vi "CreateBeamLineChargeStateNode.vi"(8 "Error In":errorcluster, 10 "Beam Line":T1={"Type"=enum."Ion Beam Analysis", "Ion"=enum."H", "Charge State"=0, "Total Source Ion Energy (kV)"=nan} {"Charge State" min=1}, 11 "DOM Document In":refnum<k20>) -> (0 "Error out":errorcluster, 2 "Beam Line Charge State Node":refnum<k20>, 3 "DOM Document Out":refnum<k20>)   [LabVIEW 2012]
uses:
  BeamLine.ctl
  BeamLineType.ctl
  BeamLineIon.ctl
  <resource>/objmgr/DOMUserDefRef.rc
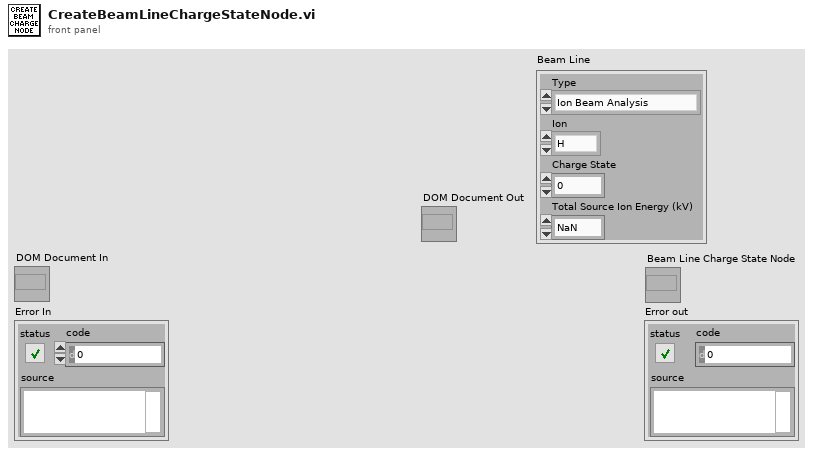
[diagram p1: front panel]
types:
  T1 = typedef "BeamLine.ctl" = cluster{"Type":T2, "Ion":T3, "Charge State":u8, "Total Source Ion Energy (kV)":dbl}
  T2 = typedef "BeamLineType.ctl" = enum16{"Ion Beam Analysis", "Auxiliary", "Radiation Damage"}
  T3 = typedef "BeamLineIon.ctl" = enum16{"H", "He", "C", "Fe", "Ni", "Pt", "Si", "Ag", "Au"}
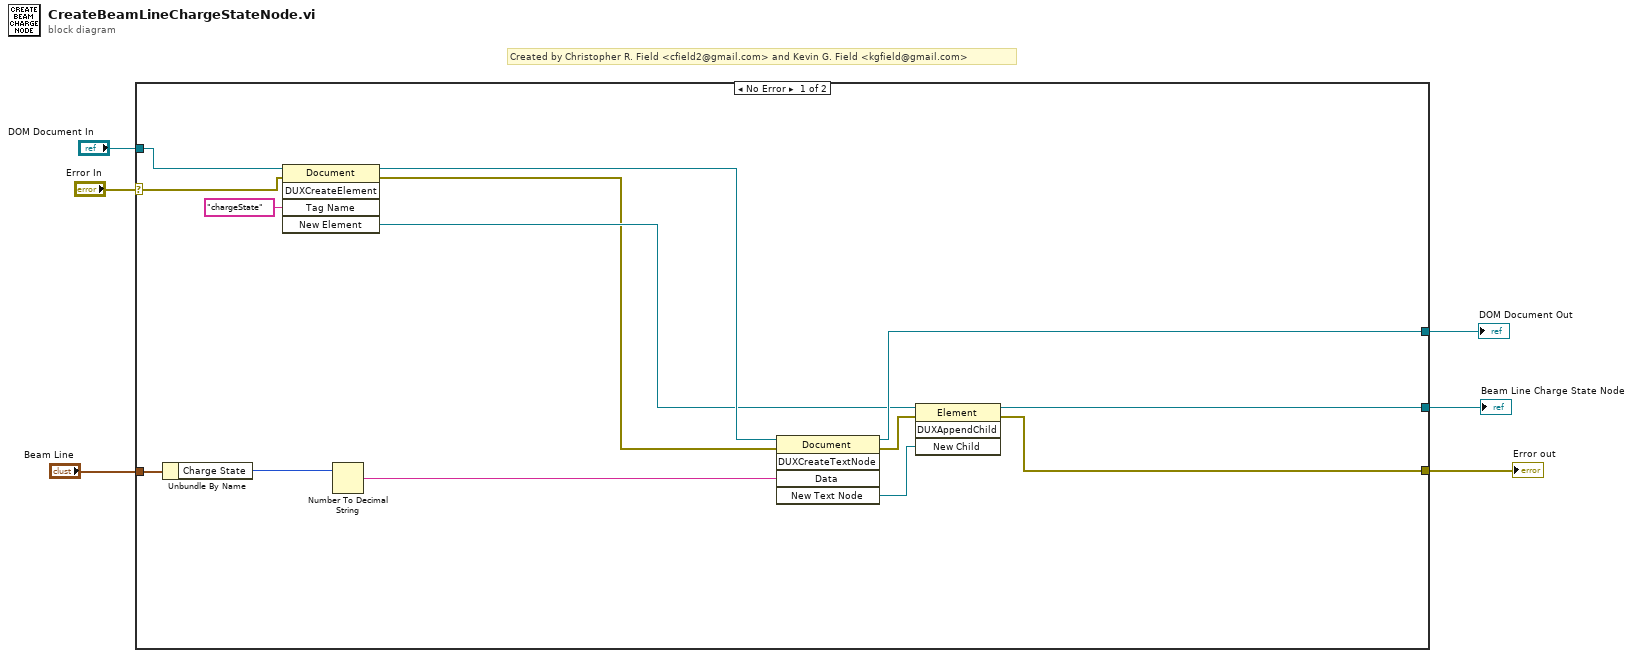
[diagram p0: block diagram]
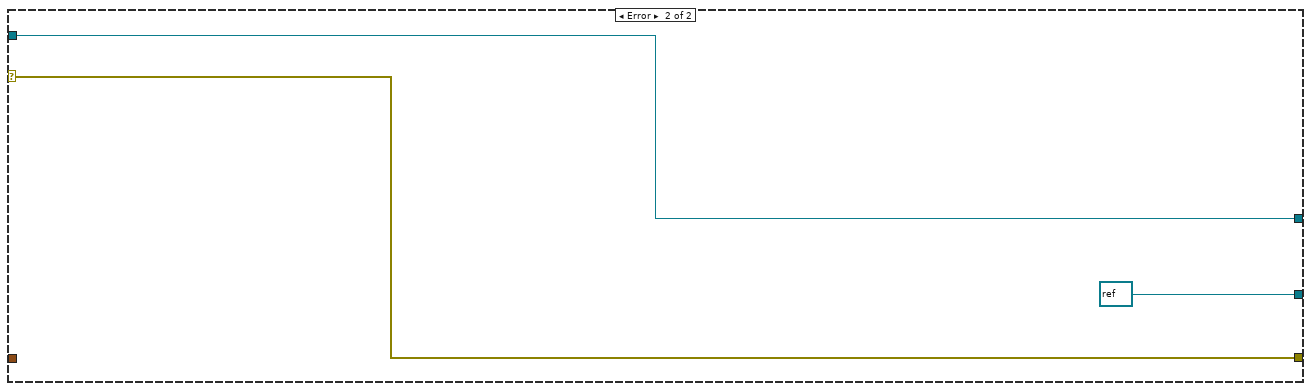
[diagram p2: hidden frame]
diagram:
  # "Created by Christopher R. Field <cfield2@gmail.com> and Kevin G. Field <kgfield@gmail.com>"
  n1 = case shown="No Error" "Error In" {
    selector: "Error In" -> [w13 w22]
    tunnel: "DOM Document In" -> [w20 w23]
    tunnel: [w19 refnum<k20> refnum ("Operator Node 2")] -> w5
    tunnel: [w18 w22] -> w4
    tunnel: "Beam Line" -> [w14 _]
    tunnel: [w12 w23] -> w2
    frame No Error {
      n2 = Unbundle By Name(w14) -> ("Charge State"=w8:u8)
      n3 = invoke class="Document" method="DUXCreateElement"(reference=w20, error in=w13, "Tag Name"="chargeState") -> (reference out=w11:refnum<k20>, error out=w9:errorcluster, "New Element"=w10:refnum<k20>)  [unwired: 2 in, 2 out]
      n4 = Number To Decimal String(number=w8) -> (decimal integer string=w7:string)  [unwired: 1 in]
      n5 = invoke class="Document" method="DUXCreateTextNode"(reference=w11, error in=w9, "Data"=w7) -> (reference out=w12:refnum<k20>, error out=w16:errorcluster, "New Text Node"=w15:refnum<k20>)  [unwired: 2 in, 2 out]
      n6 = invoke class="Element" method="DUXAppendChild"(reference=w10, error in=w16, "New Child"=w15) -> (reference out=w19:refnum<k20>, error out=w18:errorcluster)  [unwired: 1 in, 2 out]
    }
    frame Error {
    }
  }
  "Beam Line Charge State Node" <- w5
  "Error out" <- w4
  "DOM Document Out" <- w2
